vi "File Format Converter.vi"(8 "Error In":errorcluster, 10 "Configuration":T1={"New start time"=nan, "New end time"=nan, "Output file format"=enum."ASCII", "Save ASCII column names"=TRUE, "Prepend binary array size"=FALSE, "buffer size (-1: all)"=100000, "Channels"=[], "Group"="p", "New dt"=nan, "igorify column names"=TRUE, "eliminate spaces in col name"=TRUE} {"buffer size (-1: all)" format="%.0p"; "New start time" format="%#_10p"}, 11 "File":path=path "/Users/arkadyshekhter/Library/CloudStorage/Dropbox/shared_Ali/nanocal-March2020 - RuCl3/March_2020/030720/m003_030720.tdms") -> (0 "Error Out":errorcluster, 2 "New file out":path=path "/Users/arkadyshekhter/Library/CloudStorage/Dropbox/shared_Ali/nanocal-March2020 - RuCl3/March_2020/030720/m003_030720.dat", 3 "File out":path=path "/Users/arkadyshekhter/Library/CloudStorage/Dropbox/shared_Ali/nanocal-March2020 - RuCl3/March_2020/030720/m003_030720.tdms")   [LabVIEW 2021]
uses:
  Format Converter Configuration.ctl
  <vilib>/Utility/file.llb/Write Delimited Spreadsheet (DBL).vi
panel:
  out "Filename without extension":string="m003_030720"
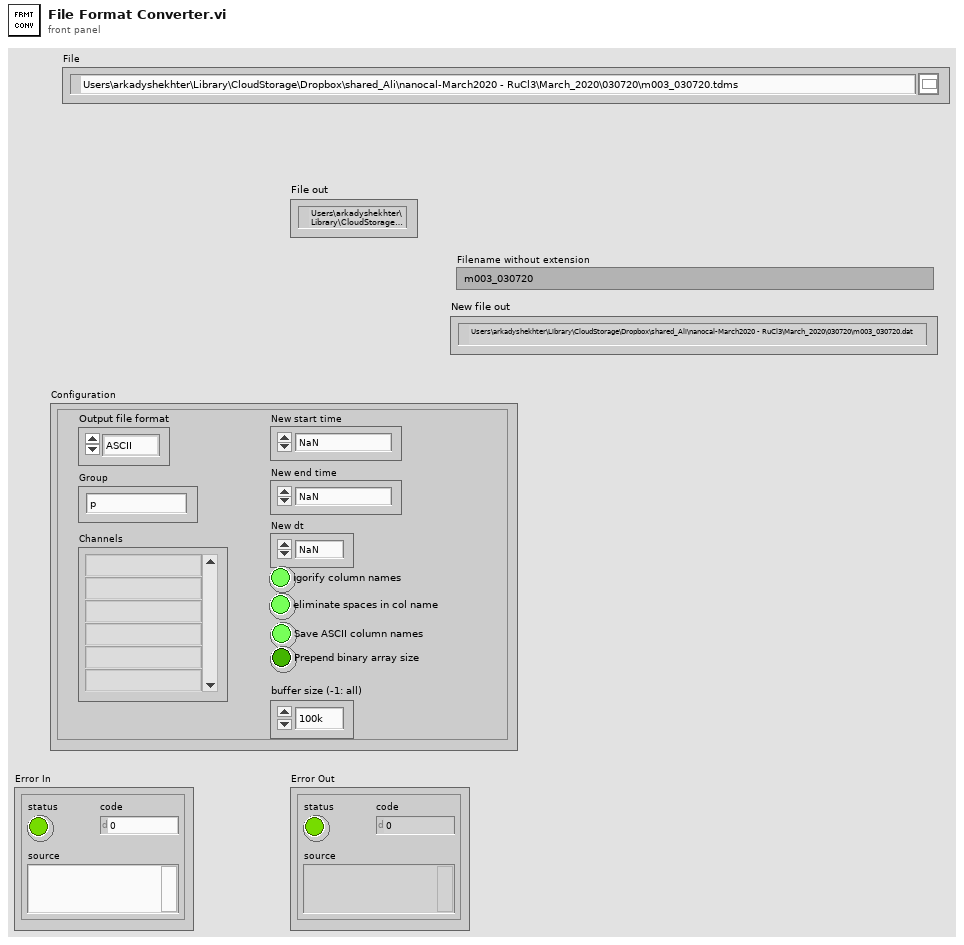
[diagram p1: front panel]
types:
  T1 = typedef "Format Converter Configuration.ctl" = cluster{"New start time":dbl, "New end time":dbl, "Output file format":enum16{"ASCII", "BINARY", "TDMS"}, "Save ASCII column names":bool, "Prepend binary array size":bool, "buffer size (-1: all)":i64, "Channels":string[], "Group":string, "New dt":dbl, "igorify column names":bool, "eliminate spaces in col name":bool}
  T2 = enum16{"open", "open or create", "create or replace", "create", "open (read-only)"}
  T3 = enum16{"open", "replace", "create", "open or create", "replace or create", "replace or create with confirmation"}
  T4 = typedef "TDMS channel info.ctl" = cluster{"t0":timestamp, "dt":dbl, "Channel length":i64}
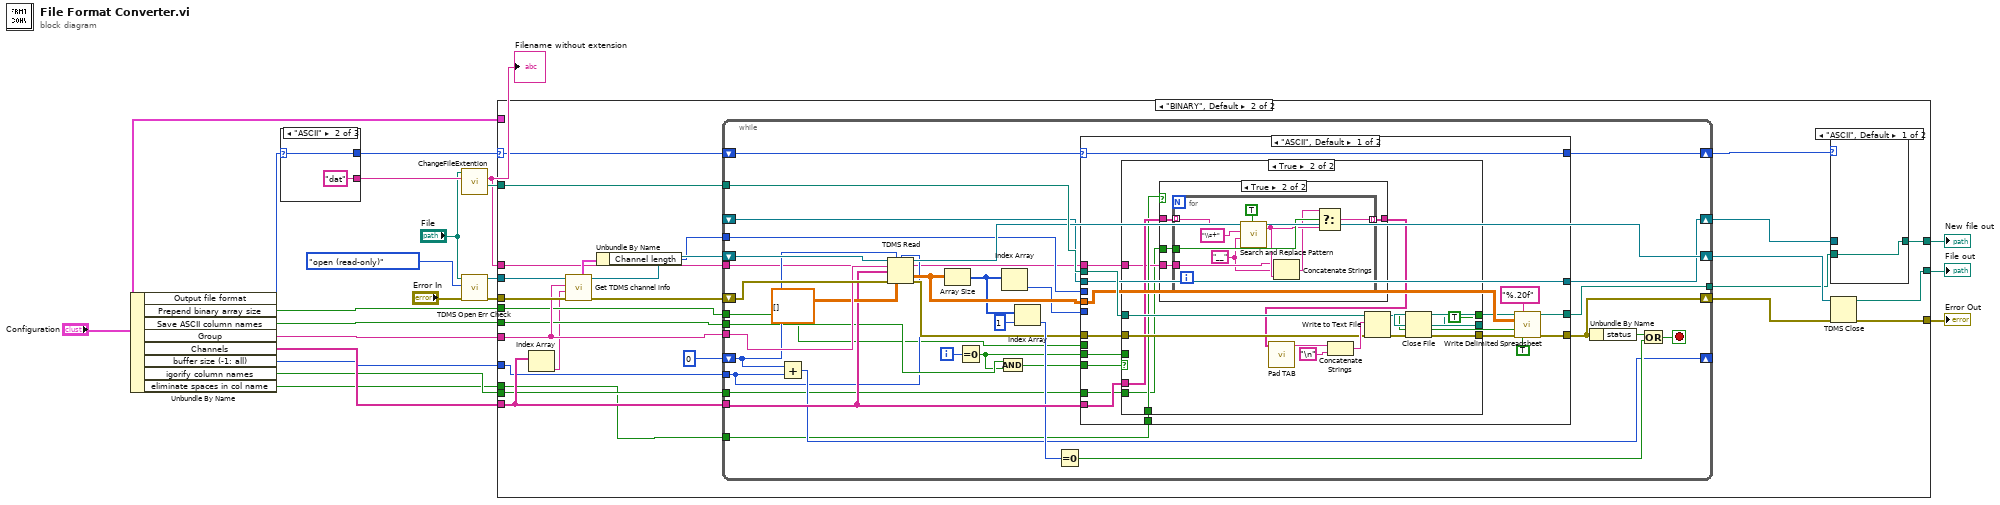
[diagram p0: block diagram]
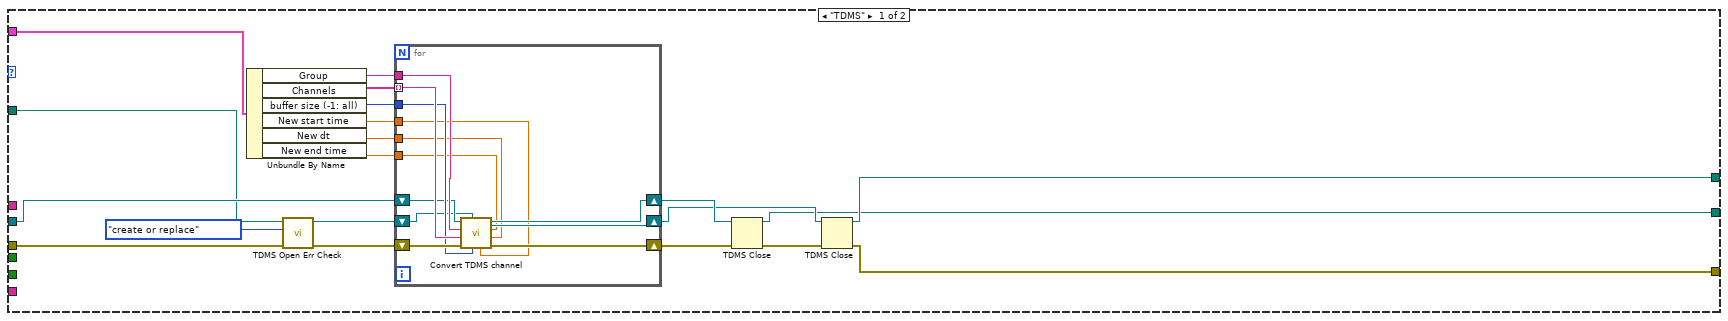
[diagram p2: hidden frame]
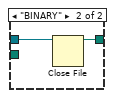
[diagram p3: hidden frame]
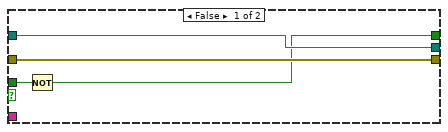
[diagram p4: hidden frame]
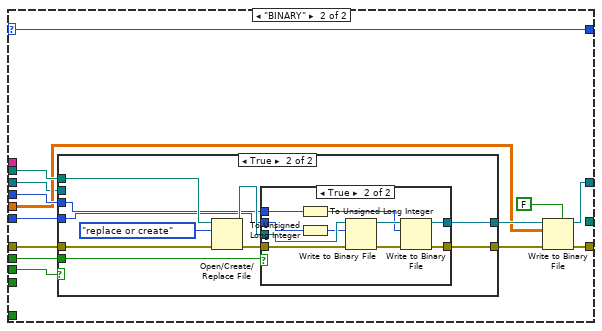
[diagram p6: hidden frame]
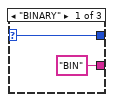
[diagram p9: hidden frame]
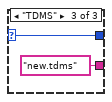
[diagram p10: hidden frame]
diagram:
  n1 = Unbundle By Name("Configuration") -> ("Output file format"=w12:enum16{"ASCII", "BINARY", "TDMS"}, "Prepend binary array size"=w14:bool, "Save ASCII column names"=w15:bool, "Group"=w17:string, "Channels"=w18:string[], "buffer size (-1: all)"=w16:i64, "igorify column names"=w3:bool, "eliminate spaces in col name"=w2:bool)
  n2 = case shown="\"ASCII\"" w12 {
    selector: w12 -> [w22 w24 w26]
    tunnel: ["BIN" ("New Extention") "dat" ("New Extention") "new.tdms" ("New Extention")] -> w21
    tunnel: [w22 w24 w26] -> w4
    frame "BINARY" {
    }
    frame "ASCII" {
    }
    frame "TDMS" {
    }
  }
  n3 = call "ChangeFileExtention.vi"("New extension"=w21, "File Path"="File") -> ("Path with new extension"=w20:path, "Filename without extension"=w1:string)  [unwired: 4 in, 4 out]
  "Filename without extension" <- w1
  n4 = call "TDMS Open Err Check.vi"("Error In"="Error In", "operation (0:open)"=T2."open (read-only)", "File Path Control"="File") -> ("Error Out"=w5:errorcluster, "tdms file out"=w6:refnum<k34>)  [unwired: 6 in, 1 out]
  n5 = case shown="\"BINARY\", Default" w4 {
    selector: w4 -> [_ w64]
    tunnel: w5 -> [w30 w85]
    tunnel: w6 -> [w47 w84]
    tunnel: w20 -> [w32 w83]
    tunnel: [w42 w82] -> w19
    tunnel: w17 -> [_ w81]
    tunnel: w18 -> [_ w80]
    tunnel: w16 -> [_ w79]
    tunnel: w15 -> [_ w78]
    tunnel: w14 -> [_ w77]
    tunnel: "Configuration" -> [w38 _]
    tunnel: [w34 w67] -> w11
    tunnel: [w33 w65] -> w10
    tunnel: w3 -> [_ w62]
    tunnel: w2 -> [_ w61]
    tunnel: w1 -> [_ w60]
    frame "TDMS" {
      n6 = Unbundle By Name(w38) -> ("Group"=w41:string, "Channels"=w40:string[], "buffer size (-1: all)"=w39:i64, "New start time"=w37:dbl, "New dt"=w36:dbl, "New end time"=w35:dbl)
      n7 = call "TDMS Open Err Check.vi"("Error In"=w30, "operation (0:open)"=T2."create or replace", "File Path Control"=w32) -> ("Error Out"=w29:errorcluster, "tdms file out"=w28:refnum<k34>)  [unwired: 6 in, 1 out]
      n8 = for {
        shift-right: [w51] -> w46
        shift-left: w29 -> [w57]
        shift-right: [w54] -> w45
        shift-left: w47 -> [w55]
        shift-right: [w52] -> w43
        shift-left: w28 -> [w53]
        tunnel: w39 -> [w56]
        tunnel: w41 -> [w59]
        tunnel: w40 -> [w58] mode=indexing
        tunnel: w37 -> [w50]
        tunnel: w36 -> [w49]
        tunnel: w35 -> [w48]
        n9 = call "Convert TDMS channel.vi"("dt"=w49, "End time"=w48, "Start time"=w50, "buffer size (-1: all)"=w56, "Output tdms ref"=w53, "Error In"=w57, "Channel name"=w58, "Group name"=w59, "Input tdms ref"=w55) -> ("Error Out"=w51:errorcluster, "Input tdms ref out"=w54:refnum<k34>, "Output tdms ref out"=w52:refnum<k34>)
      }
      n10 = TDMS Close(8:w46, 11:w45) -> (0:w44:errorcluster, 3:w33:path)
      n11 = TDMS Close(8:w44, 11:w43) -> (0:w42:errorcluster, 3:w34:path)
    }
    frame "BINARY", Default {
      n12 = Index Array(array=w80) -> (element=w72:string)  [unwired: 1 in]
      n13 = call "Get TDMS channel info.vi"("error in"=w85, "Channel name"=w72, "group name"=w81, "tdms file"=w84) -> ("error out"=w68:errorcluster, "tdms file out"=w71:refnum<k34>, "TDMS channel info"=w70:T4)  [unwired: 3 in, 2 out]
      n14 = Unbundle By Name(w70) -> ("Channel length"=w69:i64)
      n15 = while {
        tunnel: w81 -> [w121]
        tunnel: w80 -> [w118]
        tunnel: w78 -> [w111]
        tunnel: w83 -> [w117]
        shift-right: [w102] -> _
        shift-left: i64 0 -> [w114]
        shift-right: [w109] -> w74
        shift-left: w71 -> [w119]
        shift-right: [w106] -> w75
        shift-left: w68 -> [w122]
        tunnel: w69 -> [w98]
        shift-right: [w97] -> w73
        shift-left: _ -> [w96]
        tunnel: w79 -> [w95]
        tunnel: w77 -> [w94]
        tunnel: [w93] -> w66
        shift-right: [w92] -> w63
        shift-left: w64 -> [w101]
        tunnel: w62 -> [w91]
        tunnel: w61 -> [w90]
        tunnel: w60 -> [w89]
        i -> [w113]
        stop <- w105 stop-if-true
        n16 = Add(x=w114, y=w95) -> (x+y=w102:i64)
        n17 = TDMS Read(0:w119, 1:w114, 2:w95, 5:w121, 7:w118, 11:w122, 12:dbl[][] []) -> (4:w109:refnum<k34>, 10:w116:dbl[][], 15:w108:errorcluster)  [unwired: 1 in, 3 out]
        n18 = Array Size(array=w116) -> (size(s)=w100:i32[])
        n19 = Equal To 0?(x=w113) -> (x = 0?=w110:bool)
        n20 = And(x=w111, y=w110) -> (x .and. y?=w112:bool)
        n21 = Index Array(array=w100) -> (element=w99:i32)  [unwired: 1 in]
        n22 = Index Array(array=w100, index=1) -> (element=w115:i32)
        n23 = Equal To 0?(x=w115) -> (x = 0?=w104:bool)
        n24 = case shown="\"ASCII\", Default" w101 {
          selector: w101 -> [w126 w174]
          tunnel: w118 -> [w140 _]
          tunnel: w117 -> [w139 w186]
          tunnel: w116 -> [w134 w180]
          tunnel: w112 -> [w138 _]
          tunnel: w110 -> [w137 w187]
          tunnel: w108 -> [w136 w185]
          tunnel: [w129 w179] -> w106
          tunnel: w99 -> [_ w184]
          tunnel: w98 -> [_ w183]
          tunnel: [w135 w178] -> w97
          tunnel: w96 -> [w135 w177]
          tunnel: w94 -> [_ w175]
          tunnel: [w127 _] -> w93
          tunnel: [w126 w174] -> w92
          tunnel: w91 -> [w125 _]
          tunnel: w90 -> [w124 _]
          tunnel: w89 -> [w123 _]
          frame "ASCII", Default {
            n25 = case shown="True" w138 {
              tunnel: [w141 TRUE] -> w130
              tunnel: [w143 w154] -> w128
              tunnel: w140 -> [_ w149]
              tunnel: [w144 w152] -> w131
              tunnel: w136 -> [w143 w151]
              tunnel: w139 -> [w144 w150]
              tunnel: w137 -> [w142 _]
              tunnel: w125 -> [_ w145]
              tunnel: w124 -> [_ w147]
              tunnel: w123 -> [_ w146]
              frame False {
                n26 = Not(x=w142) -> (.not. x?=w141:bool)
              }
              frame True {
                n27 = case shown="True" w147 {
                  tunnel: w149 -> [w160 w164]
                  tunnel: [w160 w163] -> w148
                  tunnel: w146 -> [_ w162]
                  tunnel: w145 -> [_ w161]
                  frame False {
                  }
                  frame True {
                    n28 = for {
                      tunnel: w164 -> [w173] mode=indexing
                      tunnel: [w169] -> w163 mode=indexing
                      tunnel: w162 -> [w167]
                      tunnel: w161 -> [w170]
                      w166 = "__" ("replace string (\"\")")
                      n29 = call <vilib>:"Search and Replace Pattern.vi"("string"=w173, "regular expression (\"\")"="\\s+" ("regular expression (\"\")"), "replace string (\"\")"=w166, "replace all? (F)"=TRUE) -> ("result string"=w168:string)  [unwired: 1 in, 1 out]
                      n30 = Concatenate Strings(w167, w166, w168) -> (w165:string)
                      n31 = Select(t=w165, s=w170, f=w168) -> (s? t:f=w169:string)
                    }
                  }
                }
                n32 = call "Pad TAB.vi"("Input String Array"=w148) -> ("Output String"=w158:string)  [unwired: 10 in]
                n33 = Concatenate Strings(w158, "\n") -> (w157:string)
                n34 = Write to Text File(file (use dialog)=w150, text=w157, error in=w151) -> (refnum out=w153:refnum<file>, error out=w155:errorcluster)  [unwired: 2 out]
                n35 = Close File(refnum=w153, error in=w155) -> (path=w152:path, error out=w154:errorcluster)
              }
            }
            n36 = call-poly <vilib>:"Write Delimited Spreadsheet.vi"("file path (dialog if empty)"=w131, "format (%.3f)"="%.20f", "2D data"=w134, "append to file? (new file:F)"=w130, "error in (no error)"=w128, "transpose? (no:F)"=TRUE) -> ("new file path (Not A Path if cancelled)"=w127:path, "error out"=w129:errorcluster)  [unwired: 8 in]
          }
          frame "BINARY" {
            n37 = case shown="True" w187 {
              tunnel: w186 -> [_ w199]
              tunnel: w185 -> [w188 w198]
              tunnel: w184 -> [_ w194]
              tunnel: w183 -> [_ w193]
              tunnel: [w188 w192] -> w182
              tunnel: [w189 w191] -> w181
              tunnel: w177 -> [w189 _]
              tunnel: w175 -> [_ w190]
              frame False {
              }
              frame True {
                n38 = Open/Create/Replace File(file path (use dialog)=w199, error in=w198, operation (0:open)=T3."replace or create") -> (refnum out=w195:refnum<file>, error out=w196:errorcluster)  [unwired: 3 in, 1 out]
                n39 = case shown="True" w190 {
                  tunnel: w196 -> [w201 w211]
                  tunnel: w195 -> [w200 w210]
                  tunnel: w194 -> [_ w209]
                  tunnel: w193 -> [_ w206]
                  tunnel: [w201 w205] -> w192
                  tunnel: [w200 w204] -> w191
                  frame False {
                  }
                  frame True {
                    n40 = To Unsigned Long Integer(number=w206) -> (unsigned 32bit integer=w202:u32)
                    n41 = To Unsigned Long Integer(number=w209) -> (unsigned 32bit integer=w203:u32)
                    n42 = Write to Binary File(file (use dialog)=w210, data=w203, error in=w211) -> (refnum out=w207:refnum<file>, error out=w208:errorcluster)  [unwired: 3 in, 1 out]
                    n43 = Write to Binary File(file (use dialog)=w207, data=w202, error in=w208) -> (refnum out=w204:refnum<file>, error out=w205:errorcluster)  [unwired: 3 in, 1 out]
                  }
                }
              }
            }
            n44 = Write to Binary File(file (use dialog)=w181, data=w180, error in=w182, 5:FALSE ("prepend array or string size? (T)")) -> (refnum out=w178:refnum<file>, error out=w179:errorcluster)  [unwired: 2 in, 1 out]
          }
        }
        n45 = Unbundle By Name(w106) -> ("status"=w103:bool)
        n46 = Or(x=w103, y=w104) -> (x .or. y?=w105:bool)
      }
      n47 = case shown="\"ASCII\", Default" w63 {
        tunnel: w73 -> [_ w88]
        tunnel: [w86 w87] -> w67
        tunnel: w66 -> [w86 _]
        frame "ASCII", Default {
        }
        frame "BINARY" {
          n48 = Close File(refnum=w88) -> (path=w87:path)  [unwired: 1 in, 1 out]
        }
      }
      n49 = TDMS Close(8:w75, 11:w74) -> (0:w82:errorcluster, 3:w65:path)
    }
  }
  "Error Out" <- w19
  "File out" <- w10
  "New file out" <- w11
